vi "Get SLSC Module By Name.vi"(8 "error in (no error)":errorcluster, 10 "Name":string, 11 "SLSC Chassis":u64) -> (0 "error out":errorcluster, 1 "Found":bool, 2 "SLSC Module":u64, 3 "SLSC Chassis out":u64)   [LabVIEW 2017, in "VeriStand SLSC Scripting.lvlib"]
uses:
  VeriStand SLSC Scripting.lvlib
  NationalInstruments.VeriStand.SystemDefinitionAPI
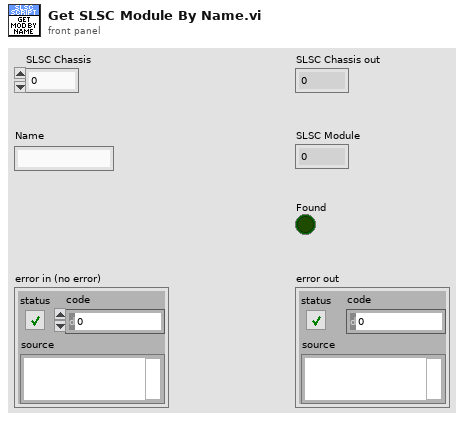
[diagram p1: front panel]
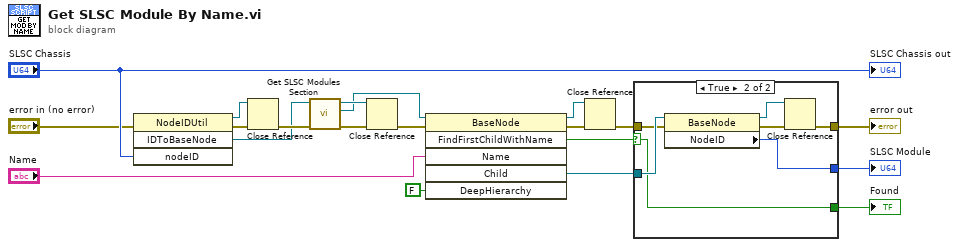
[diagram p0: block diagram]
diagram:
  n1 = invoke class="NodeIDUtil" method="IDToBaseNode"(error in="error in (no error)", "nodeID"="SLSC Chassis") -> (reference out=w19:refnum<k24>, error out=w20:errorcluster, "IDToBaseNode"=w5:refnum<k24>)  [unwired: 2 in, 1 out]
  n2 = Close Reference(reference=w19, error in (no error)=w20) -> (error out=w6:errorcluster)
  n3 = call "Get SLSC Modules Section.vi"("error in (no error)"=w6, "SLSC Chassis"=w5) -> ("error out"=w4:errorcluster, "Modules Section"=w1:refnum<k24>, "SLSC Chassis out"=w3:refnum<k24>)  [unwired: 7 in]
  n4 = Close Reference(reference=w3, error in (no error)=w4) -> (error out=w2:errorcluster)
  n5 = invoke class="BaseNode" method="FindFirstChildWithName"(reference=w1, error in=w2, "Name"="Name", "DeepHierarchy"=FALSE) -> (reference out=w10:refnum<k24>, error out=w13:errorcluster, "FindFirstChildWithName"=w9:bool, "Child"=w12:refnum<k24>)  [unwired: 2 in, 2 out]
  n6 = Close Reference(reference=w10, error in (no error)=w13) -> (error out=w11:errorcluster)
  n7 = case shown="True" w9 {
    selector: w9 -> [w21 w26]
    tunnel: [w22 w24] -> w7
    tunnel: [_ w29] -> w16
    tunnel: w12 -> [_ w28]
    tunnel: w11 -> [w22 w27]
    tunnel: [w21 w26] -> w8
    frame False {
    }
    frame True {
      n8 = property class="BaseNode"(reference=w28, error in=w27) -> (reference out=w23:refnum<k24>, error out=w25:errorcluster, "NodeID"=w29:u64)
      n9 = Close Reference(reference=w23, error in (no error)=w25) -> (error out=w24:errorcluster)
    }
  }
  "error out" <- w7
  "SLSC Module" <- w16
  "Found" <- w8
  "SLSC Chassis out" <- "SLSC Chassis"
